vi "RSZVB Set Linearity Deviation Slope.vi"(8 "error in (no error)":errorcluster {"code" format="%.0x"}, 9 "Slope (0.0 dB/MHz)":dbl format="%^.3e", 10 "Channel (1)":i32=1, 11 "VISA session":refnum<visa-resource-name>) -> (0 "error out":errorcluster {"code" format="%.0x"}, 3 "dup VISA session":refnum<visa-resource-name>)   [LabVIEW 2011]
doc: "This VI defines the slope of the regression line for the linearity deviation calculation. \n\nRemote-control command(s):\nCALCulate<Chn>:LDEViation:SLOPe"
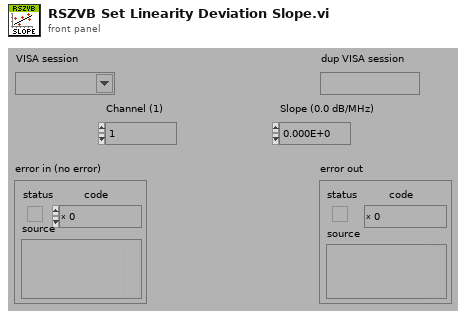
[diagram p1: front panel]
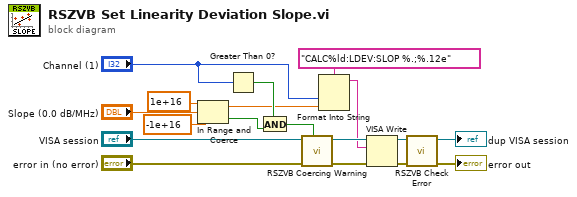
[diagram p0: block diagram]
diagram:
  n1 = In Range and Coerce(upper limit=1e+16, x="Slope (0.0 dB/MHz)", lower limit=-1e+16) -> (coerced(x)=w2:dbl, In Range?=w1:bool)
  n2 = Greater Than 0?(x="Channel (1)") -> (x > 0?=w15:bool)
  n3 = And(x=w15, y=w1) -> (x .and. y?=w14:bool)
  n4 = call "RSZVB Coercing Warning.vi"("In Range?"=w14, "error in (no error)"="error in (no error)", "VISA session"="VISA session") -> ("error out"=w16:errorcluster, "dup VISA session"=w13:refnum<visa-resource-name>)  [unwired: 7 in]
  n5 = Format Into String(format string="CALC%ld:LDEV:SLOP %.;%.12e", "Channel (1)", w2) -> (resulting string=w12:string)  [unwired: 2 in, 1 out]
  n6 = VISA Write(VISA resource name=w13, write buffer=w12, error in (no error)=w16) -> (VISA resource name out=w17:refnum<visa-resource-name>, error out=w18:errorcluster)  [unwired: 1 out]
  n7 = call "RSZVB Check Error.vi"("error in (no error)"=w18, "VISA session"=w17) -> ("error out"=→"error out":errorcluster, "dup VISA session"=→"dup VISA session":refnum<visa-resource-name>)  [unwired: 8 in]
